vi "Face Corridor.vi"(2 "Starting Position":T4=enum."Far Right", 3 "Command Info In":T1) -> (10 "Command Info Out":T1)   [LabVIEW 2017]
uses:
  <vilib>/Rock Robotics/WPI/Framework/Command Status Info.ctl
  <vilib>/Rock Robotics/WPI/Framework/Completion Status.ctl
  <vilib>/Rock Robotics/WPI/Framework/Completion Notifier.ctl
  Support Code/Starting Position.ctl
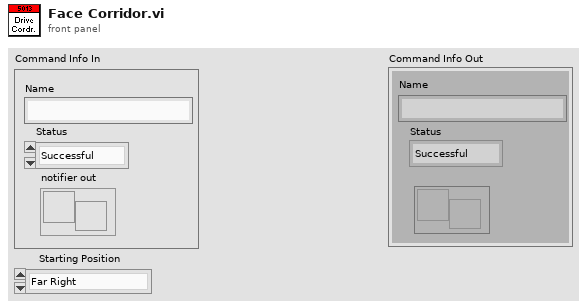
[diagram p1: front panel]
types:
  T1 = typedef "Command Status Info.ctl" = cluster{"Name":string, "Status":T2, "notifier out":T3}
  T2 = typedef "Completion Status.ctl" = enum16{"Successful", "Aborted", "Incomplete"}
  T3 = typedef "Completion Notifier.ctl" = refnum<notifier>
  T4 = typedef "Starting Position.ctl" = enum16{"Far Left", "Right", "Far Right"}
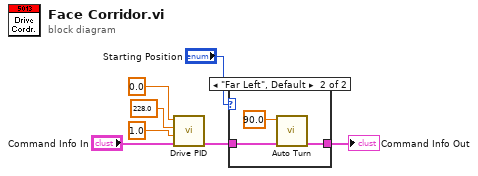
[diagram p0: block diagram]
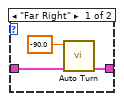
[diagram p2: hidden frame]
diagram:
  n1 = call "Drive PID.vi"("Command Info In"="Command Info In", "Speed"=1.0, "Distance"=228.0, "Target Angle"=0.0) -> ("Command Info Out"=w2:T1)  [unwired: 7 in]
  n2 = case shown="\"Far Left\", Default" "Starting Position" {
    tunnel: w2 -> [w9 w13]
    tunnel: [w8 w11] -> w1
    frame "Far Right" {
      n3 = call "Auto Turn.vi"("Command Info In"=w9, "Target Angle"=-90.0) -> ("Command Info Out"=w8:T1)  [unwired: 9 in]
    }
    frame "Far Left", Default {
      n4 = call "Auto Turn.vi"("Command Info In"=w13, "Target Angle"=90.0) -> ("Command Info Out"=w11:T1)  [unwired: 9 in]
    }
  }
  "Command Info Out" <- w1
